vi "Read Context.vi"(8 "error in":errorcluster, 11 "State in":refnum<class "B State.lvclass">) -> (0 "error out":errorcluster, 2 "Context":refnum<class "State Pattern.lvclass">, 3 "State out":refnum<class "B State.lvclass">)   [LabVIEW 2021, in "Context.lvlib" / "B State.lvclass"]
uses:
  B State.lvclass
  State Pattern/State Pattern/State Pattern.lvclass
  B State.lvclass/B State.ctl
  Context/Context.lvclass
  C:/PPLs/Design-Patterns/State Pattern/State Pattern/State Pattern/State Pattern.lvclass
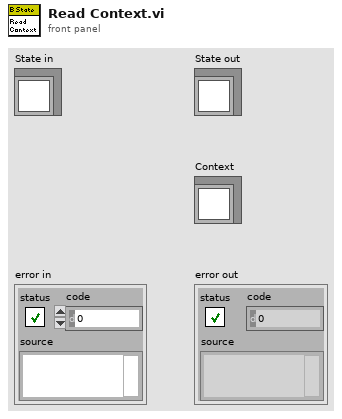
[diagram p1: front panel]
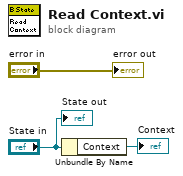
[diagram p0: block diagram]
diagram:
  n1 = Unbundle By Name("State in") -> ("Context"=→"Context":refnum<class "Context.lvclass">)
  "error out" <- "error in"
  "State out" <- "State in"
